vi "Close-GUI.vi"(8 "error in (no error)":errorcluster, 11 "Main VI":refnum<vi>) -> (0 "error out":errorcluster)   [LabVIEW 2013, in "SLMControl.lvlib" / "SC-Main.lvclass"]
uses:
  SC-Main.lvclass
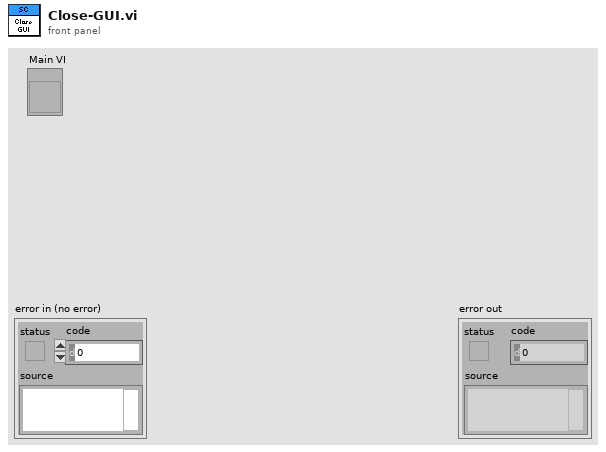
[diagram p1: front panel]
types:
  T1 = enum32{"invalid app kind", "Development System", "Run Time System", "Student Edition", "Embedded LabVIEW", "Evaluation", "Custom"}
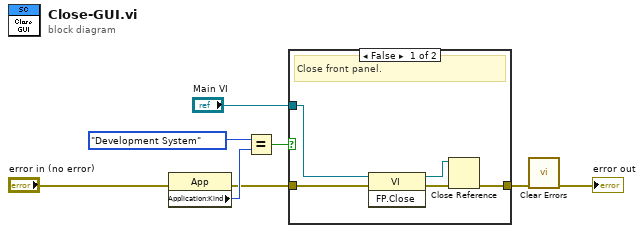
[diagram p0: block diagram]
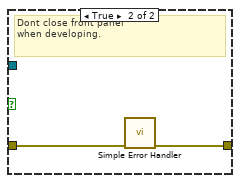
[diagram p2: hidden frame]
diagram:
  n1 = property on="Property Node" class="App"(error in="error in (no error)") -> (error out=w3:errorcluster, "Application:Kind"=w6:T1)  [unwired: 1 in, 1 out]
  n2 = Equal?(x=T1."Development System" ("y"), y=w6) -> (x = y?=w4:bool)
  n3 = case shown="False" w4 {
    tunnel: w3 -> [w13 w15]
    tunnel: [w10 w14] -> w2
    tunnel: "Main VI" -> [w12 _]
    frame False {
      # "Close front panel."
      n4 = invoke class="VI" method="FP.Close"(reference=w12, error in=w13) -> (reference out=w9:refnum<vi>, error out=w11:errorcluster)  [unwired: 1 in, 1 out]
      n5 = Close Reference(reference=w9, error in (no error)=w11) -> (error out=w10:errorcluster)
    }
    frame True {
      # "Dont close front panel\nwhen developing."
      n6 = call <vilib>:"Simple Error Handler.vi"("error in (no error)"=w15) -> ("error out"=w14:errorcluster)  [unwired: 4 in, 4 out]
    }
  }
  n7 = call <vilib>:"Clear Errors.vi"("error in (no error)"=w2) -> ("error out"=→"error out":errorcluster)  [unwired: 6 in]
